vi "Contour_Manual.vi"(4 "Properties":T1={"Label Contours"=FALSE, "Line"={"Style"=enum."Automatic", "Color"=2147483647, "Width"=nan}, "Display"={"Alpha"=nan, "Z Order"=nan}} {"Line"."Color" items=["Automatic"=2147483647, "Black"=0, "White"=16777215, "Red"=16711680, "Green"=2263842, "Blue"=255, "Cyan"=65535, "Magenta"=16711935, "Yellow"=16776960]}, 5 "Levels":dbl[](array[numeric]), 7 "Z Data":dbl[][](array[numeric]), 8 "error in (no error)":errorcluster, 9 "Y Coordinates":dbl[](array[numeric]), 10 "X Coordinates":dbl[](array[numeric]), 11 "Plot ID":T6 format="%x") -> (0 "error out":errorcluster, 3 "Plot ID Out":T6 format="%x")   [LabVIEW 2013, in "Advanced Plotting Toolkit.lvlib"]
doc: "Make a 2D contour plot, with explicitly specified contour levels."
uses:
  Advanced Plotting Toolkit.lvlib
  typedefs/PlotID.ctl
  ContourProperties.ctl
  properties/Line.ctl
  properties/Line_Style.ctl
  typedefs/PlotColor.ctl
  properties/Display.ctl
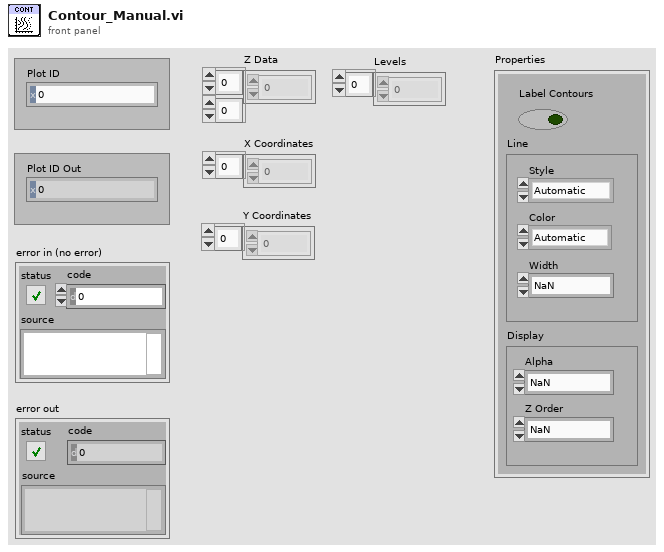
[diagram p1: front panel]
types:
  T1 = typedef "Advanced Plotting Toolkit.lvlib/ContourProperties.ctl" = cluster{"Label Contours":bool, "Line":T2, "Display":T5}
  T2 = typedef "Advanced Plotting Toolkit.lvlib/Line.ctl" = cluster{"Style":T3, "Color":T4, "Width":sgl}
  T3 = typedef "Advanced Plotting Toolkit.lvlib/Line_Style.ctl" = enum16{"Automatic", "Solid", "Dashed", "Dotted", "Dash-dot", "Invisible"}
  T4 = typedef "Advanced Plotting Toolkit.lvlib/PlotColor.ctl" = u32
  T5 = typedef "Advanced Plotting Toolkit.lvlib/Display.ctl" = cluster{"Alpha":dbl, "Z Order":dbl}
  T6 = typedef "Advanced Plotting Toolkit.lvlib/PlotID.ctl" = i32
  T7 = typedef "Advanced Plotting Toolkit.lvlib/KeyValue.ctl" = cluster{"Key":string, "Value":string}
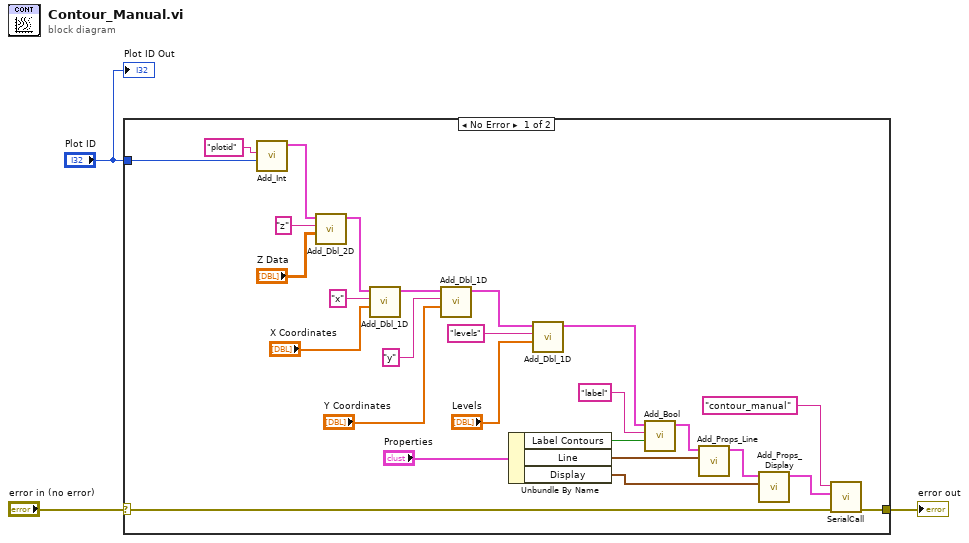
[diagram p0: block diagram]
diagram:
  n1 = case shown="No Error" "error in (no error)" {
    selector: "error in (no error)" -> [w19 w30]
    tunnel: "Plot ID" -> [w17 _]
    tunnel: [w18 w30] -> w1
    frame No Error {
      n2 = call "Add_Int.vi"("Value"=w17, "Key"="plotid") -> ("Keyword Array Out"=w25:T7[])  [unwired: 9 in]
      n3 = call "Add_Dbl_2D.vi"("Value"="Z Data", "Key"="z", "Keyword Array"=w25) -> ("Keyword Array Out"=w24:T7[])  [unwired: 8 in]
      n4 = call "Add_Dbl_1D.vi"("Value"="X Coordinates", "Key"="x", "Keyword Array"=w24) -> ("Keyword Array Out"=w23:T7[])  [unwired: 8 in]
      n5 = call "Add_Dbl_1D.vi"("Value"="Y Coordinates", "Key"="y", "Keyword Array"=w23) -> ("Keyword Array Out"=w8:T7[])  [unwired: 8 in]
      n6 = Unbundle By Name("Properties") -> ("Label Contours"=w10:bool, "Line"=w12:T2, "Display"=w11:T5)
      n7 = call "Add_Dbl_1D.vi"("Value"="Levels", "Key"="levels", "Keyword Array"=w8) -> ("Keyword Array Out"=w5:T7[])  [unwired: 8 in]
      n8 = call "Add_Bool.vi"("Value"=w10, "Key"="label", "Keyword Array"=w5) -> ("Keyword Array Out"=w9:T7[])  [unwired: 8 in]
      n9 = call "Add_Props_Line.vi"("Line"=w12, "Keyword Array"=w9) -> ("Keyword Array Out"=w4:T7[])  [unwired: 9 in]
      n10 = call "Add_Props_Display.vi"("Display"=w11, "Keyword Array"=w4) -> ("Keyword Array Out"=w13:T7[])  [unwired: 9 in]
      n11 = call "SerialCall.vi"("error in (no error)"=w19, "data"=w13, "Resource"="contour_manual") -> ("error out"=w18:errorcluster)  [unwired: 7 in, 1 out]
    }
    frame Error {
    }
  }
  "error out" <- w1
  "Plot ID Out" <- "Plot ID"
